vi "Calculate Mean.vi"(11 "Statistics in":refnum<class "JSON Value.lvclass">) -> (3 "Mean":refnum<class "JSON Value.lvclass">)   [LabVIEW 2020, in "Library Commun.lvlib" / "JSON Running Mean.lvclass"]
uses:
  JSON Running Mean.lvclass
  JSON Value/JSON Value.lvclass
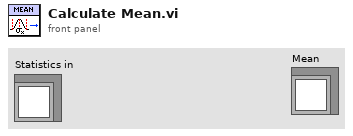
[diagram p1: front panel]
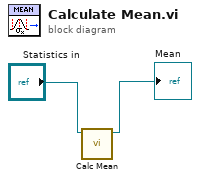
[diagram p0: block diagram]
diagram:
  n1 = call-dynamic "Calc Mean.vi"("JSON Value In"="Statistics in") -> ("JSON Value"=→"Mean":refnum<class "JSON Value.lvclass">)  [unwired: 10 in]
